vi "State PSOC Simple Serial.vi"() -> ()   [LabVIEW 2019]
uses:
  Serial - Settings.ctl
  State Simple Serial.ctl
  <vilib>/Platform/TimedLoop/XDataNode/timing_clust.ctl
  <vilib>/Platform/TimedLoop/XDataNode/nitl_modes.ctl
  <vilib>/Platform/TimedLoop/XDataNode/wakeup.ctl
  <vilib>/Instr/_visa.llb/VISA Configure Serial Port (Instr).vi
  <vilib>/platform/TimedLoop/XDataNode/XDataNode.xnode
  <vilib>/Platform/TimedLoop/XDataNode/XDNodeRunTimeDep.lvlib
panel:
  in  "?":bool
  out "unsigned byte array":u8[](array[numeric])
  out "bytes read":u32
  out "Response":string
  in  "Serial Settings":T1={"baud rate"=115200, "data bits"=8, "parity"=enum."None", "stop bits"=10, "flow control"=0} {"flow control" items=["None"=0, "XON/XOFF"=1, "RTS/CTS"=2, "DTR/DSR"=4]; "stop bits" items=["1.0"=10, "1.5"=15, "2.0"=20]; "data bits" min=5 max=8 step=1; "baud rate" items=["75"=75, "110"=110, "134"=134, "150"=150, "300"=300, "600"=600, "1200"=1200, "1800"=1800, "2400"=2400, "4800"=4800, "7200"=7200, "9600"=9600, "14400"=14400, "19200"=19200, "28800"=28800, "38400"=38400, "56000"=56000, "57600"=57600, "115200"=115200, "128000"=128000, "230400"=230400]}
  in  "delay before read (ms)":u32=500
  in  "VISA resource name":refnum<visa-resource-name>="COM1"
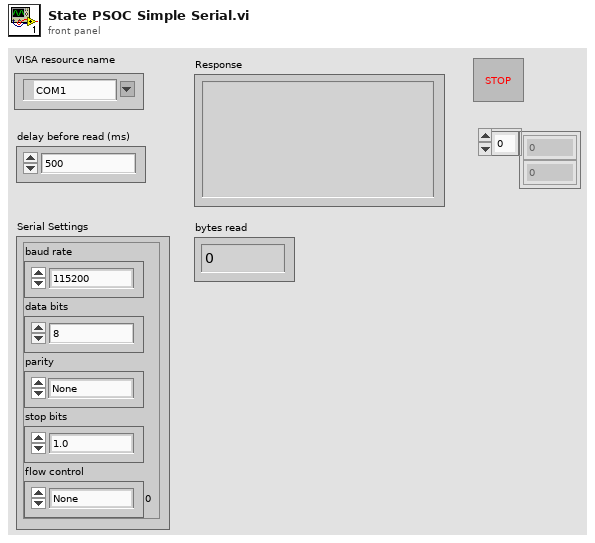
[diagram p1: front panel]
types:
  T1 = typedef "Serial - Settings.ctl" = cluster{"baud rate":u32, "data bits":u16, "parity":enum16{"None", "Odd", "Even", "Mark", "Space"}, "stop bits":u16, "flow control":u16}
  T2 = typedef "State Simple Serial.ctl" = enum16{"Open", "Write", "Wait", "Read", "Close"}
  T3 = typedef "XDNodeRunTimeDep.lvlib/timing_clust.ctl" = cluster{"Expected End [f-1]":u64, "Actual End [f-1]":u64, "Finished Late? [f-1]":bool, "Expected End [i-1]":u64, "Actual End [i-1]":u64, "Finished Late? [i-1]":bool, "Expected Start [i]":u64, "Actual Start [i]":u64, "Expected Start [f]":u64, "Actual Start [f]":u64, "Source Name":string, "Structure Name":string, "Period":i64, "Deadline":i64, "Offset":i64, "Start":i64, "Priority":i32, "Timeout":i32, "Mode":T4, "Wakeup Reason":T5, "Error":errorcluster, "Source Type":string, "Secondary Source Type":string, "Global End Time":u64, "Global Start Time":u64, "Frame Duration":u64, "Iteration Duration":u64, "Assigned CPU":i32, "I/O Scan Engine Mode":u32}
  T4 = typedef "XDNodeRunTimeDep.lvlib/nitl_modes.ctl" = enum32{"No Change", "Process missed periods, maintain original phase", "Discard missed periods, maintain original phase", "Process missed periods, ignore original phase", "Discard missed periods, ignore original phase"}
  T5 = typedef "XDNodeRunTimeDep.lvlib/wakeup.ctl" = enum32{"Normal", "Aborted", "Asynchronous wakeup", "Timing source error", "Timed loop error", "Timeout"}
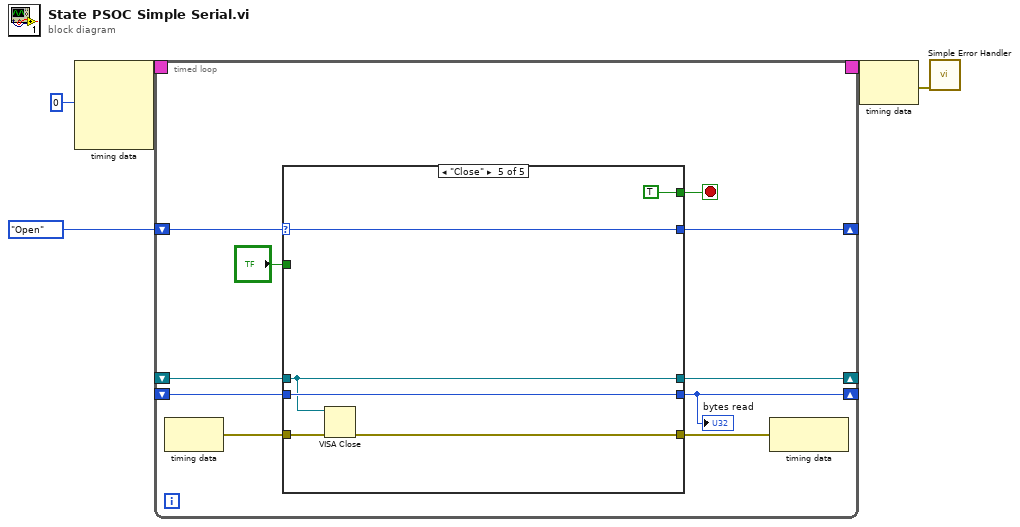
[diagram p0: block diagram]
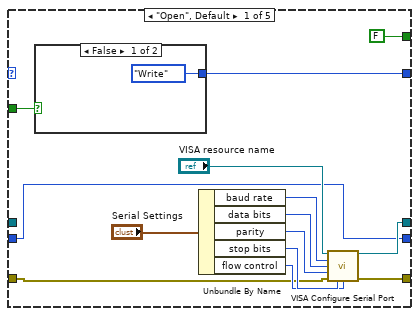
[diagram p2: hidden frame]
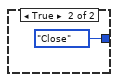
[diagram p3: hidden frame]
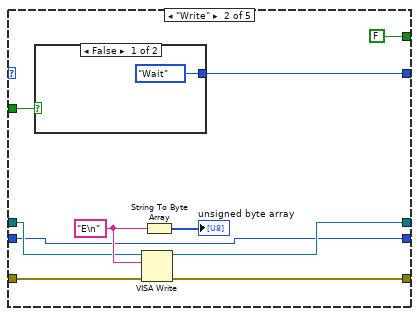
[diagram p4: hidden frame]
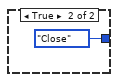
[diagram p5: hidden frame]
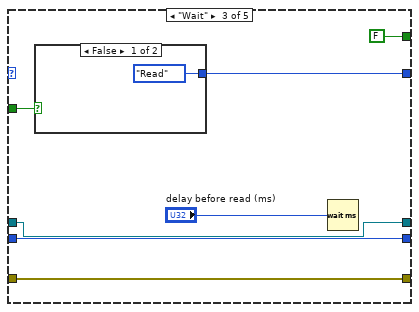
[diagram p6: hidden frame]
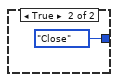
[diagram p7: hidden frame]
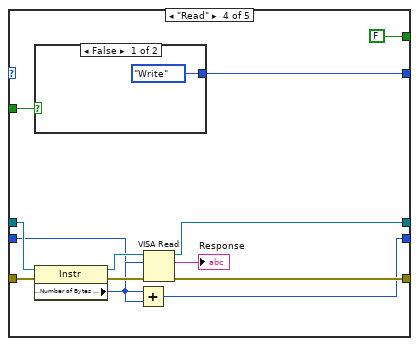
[diagram p8: hidden frame]
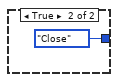
[diagram p9: hidden frame]
diagram:
  n1 = node-c288(i64 0 ("Period")) -> (w5:T3)  [unwired: 3 in]
  n2 = timed-loop {
    timing: w5 -> [_]
    timing-out: [_] -> w4
    shift-right: [w13] -> _
    shift-left: State_Simple_Serial."Open" -> [w15]
    shift-right: [w9] -> _
    shift-left: _ -> [w8]
    shift-right: [w7] -> _
    shift-left: _ -> [w6]
    stop <- w11 stop-if-true
    n3 = node-c288() -> (w14:errorcluster)  [unwired: 1 in]
    n4 = case shown="\"Close\"" w15 {
      selector: w15 -> [_ _ _ _ w72]
      tunnel: w14 -> [w23 w41 w49 w62 w70]
      tunnel: [w20 w37 w47 w59 w72] -> w13
      tunnel: [w22 w39 w49 w60 w69] -> w12
      tunnel: [FALSE ("Boolean") FALSE ("Boolean") FALSE ("Boolean") FALSE ("Boolean") TRUE ("Boolean")] -> w11
      tunnel: "?" -> [w19 w36 w46 w58 _]
      tunnel: [w17 w34 w45 w56 w68] -> w9
      tunnel: w8 -> [_ w35 w45 w57 w68]
      tunnel: [w16 w32 w44 w54 w71] -> w7
      tunnel: w6 -> [w16 w32 w44 w53 w71]
      frame "Open", Default {
        n5 = case shown="False" w19 {
          tunnel: [State_Simple_Serial."Write" State_Simple_Serial."Close"] -> w20
          frame False {
          }
          frame True {
          }
        }
        n6 = Unbundle By Name("Serial Settings") -> ("baud rate"=w28:u32, "data bits"=w27:u16, "parity"=w26:enum16{"None", "Odd", "Even", "Mark", "Space"}, "stop bits"=w25:u16, "flow control"=w24:u16)
        n7 = call-poly "VISA Configure Serial Port"("VISA resource name"="VISA resource name", "baud rate (9600)"=w28, "data bits (8)"=w27, "parity (0:none)"=w26, "error in (no error)"=w23, "stop bits (10: 1 bit)"=w25, "flow control (0:none)"=w24) -> ("VISA resource name out"=w17:refnum<visa-resource-name>, "error out"=w22:errorcluster)  [unwired: 2 in, 5 out]
      }
      frame "Write" {
        w40 = "E\n" ("Command")
        n8 = case shown="False" w36 {
          tunnel: [State_Simple_Serial."Wait" State_Simple_Serial."Close"] -> w37
          frame False {
          }
          frame True {
          }
        }
        n9 = VISA Write(VISA resource name=w35, write buffer=w40, error in (no error)=w41) -> (VISA resource name out=w34:refnum<visa-resource-name>, error out=w39:errorcluster)  [unwired: 1 out]
        n10 = String To Byte Array(string=w40) -> (unsigned byte array=→"unsigned byte array":u8[])
      }
      frame "Wait" {
        n11 = case shown="False" w46 {
          tunnel: [State_Simple_Serial."Read" State_Simple_Serial."Close"] -> w47
          frame False {
          }
          frame True {
          }
        }
        n12 = Wait (ms)(milliseconds to wait="delay before read (ms)") -> ()  [unwired: 1 out]
      }
      frame "Read" {
        n13 = case shown="False" w58 {
          tunnel: [State_Simple_Serial."Write" State_Simple_Serial."Close"] -> w59
          frame False {
          }
          frame True {
          }
        }
        n14 = property class="Instr"(reference=w57, error in=w62) -> (reference out=w63:refnum<visa-resource-name>, error out=w64:errorcluster, "Serial Settings:Number of Bytes at Serial Port"=w55:u32)
        n15 = Add(x=w55, y=w53) -> (x+y=w54:u32)
        n16 = VISA Read(VISA resource name=w63, byte count=w55, error in (no error)=w64) -> (VISA resource name out=w56:refnum<visa-resource-name>, read buffer=→"Response":string, error out=w60:errorcluster)  [unwired: 1 out]
      }
      frame "Close" {
        n17 = VISA Close(VISA resource name=w68, error in (no error)=w70) -> (error out=w69:errorcluster)
      }
    }
    "bytes read" <- w7
    n18 = node-c288(w12) -> ()  [unwired: 1 out]
  }
  n19 = node-c288(w4) -> (w2:errorcluster)
  n20 = call <vilib>:"Simple Error Handler.vi"("error in (no error)"=w2) -> ()  [unwired: 1 in, 8 out]
